vi "LINC COSMOS Item.vi"(5 "ignore":bool, 6 "ID?":bool, 8 "error in (no error)":errorcluster, 9 "packet fields":T1, 10 "packet index":i32, 11 "packets in":T2[](array[typedef])) -> (0 "error out":errorcluster, 2 "item index":i32, 3 "packets out":T2[](array[typedef]))   [LabVIEW 2018, in "STEPkgDriver_LINC.lvlib"]
uses:
  STEPkgDriver_LINC.lvlib
  LINC Format Prototype.ctl
  LINC Packet.ctl
  LINC Packet Fields.ctl
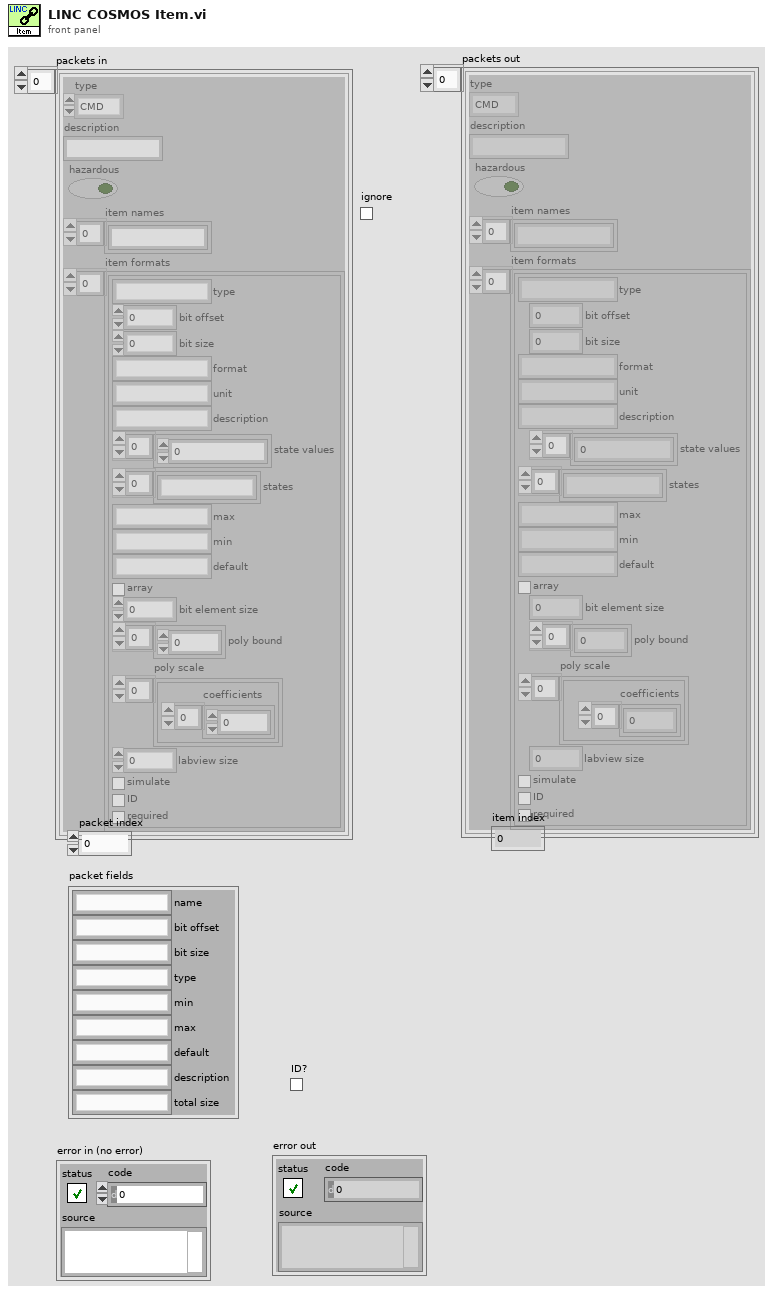
[diagram p1: front panel]
types:
  T1 = typedef "STEPkgDriver_LINC.lvlib/LINC Packet Fields.ctl" = cluster{"name":string, "bit offset":string, "bit size":string, "type":string, "min":string, "max":string, "default":string, "description":string, "total size":string}
  T2 = typedef "STEPkgDriver_LINC.lvlib/LINC Packet.ctl" = cluster{"type":enum16{"CMD", "TLM"}, "description":string, "hazardous":bool, "item names":string[], "item formats":T3[]}
  T3 = typedef "STEPkgDriver_LINC.lvlib/LINC Format Prototype.ctl" = cluster{"type":string, "bit offset":i32, "bit size":i32, "format":string, "unit":string, "description":string, "state values":i64[], "states":string[], "max":string, "min":string, "default":string, "array":bool, "bit element size":i32, "poly bound":dbl[], "poly scale":cluster{"coefficients":dbl[]}[], "labview size":i32, "simulate":bool, "ID":bool, "required":bool}
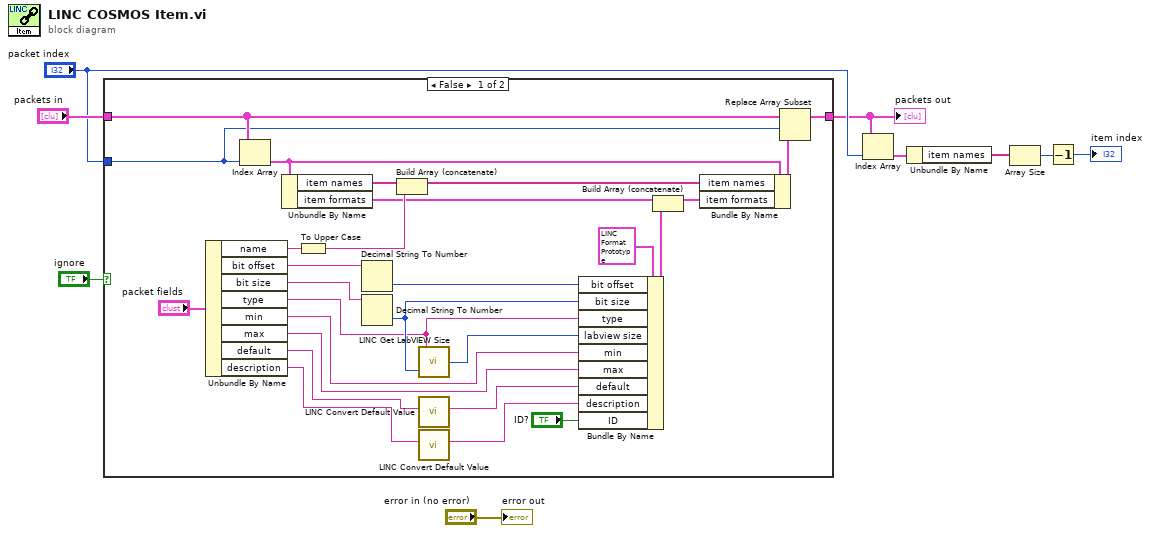
[diagram p0: block diagram]
diagram:
  n1 = case shown="False" "ignore" {
    tunnel: "packets in" -> [w21 w37]
    tunnel: [w20 w37] -> w5
    tunnel: "packet index" -> [w10 _]
    frame False {
      n2 = Unbundle By Name("packet fields") -> ("name"=w17:string, "bit offset"=w16:string, "bit size"=w15:string, "type"=w14:string, "min"=w13:string, "max"=w12:string, "default"=w11:string, "description"=w29:string)
      n3 = Index Array(array=w21, index=w10) -> (element=w27:T2)
      n4 = Unbundle By Name(w27) -> ("item names"=w25:string[], "item formats"=w22:T3[])
      n5 = To Upper Case(1:w17) -> (0:w32:string)
      n6 = Decimal String To Number(string=w16) -> (number=w33:i32)  [unwired: 2 in, 1 out]
      n7 = Decimal String To Number(string=w15) -> (number=w31:i32)  [unwired: 2 in, 1 out]
      n8 = Build Array (concatenate)(w25, w32) -> (w24:string[])
      n9 = call "LINC Get LabVIEW Size.vi"("bit size"=w31, "type"=w14) -> ("labview size"=w30:i32)
      n10 = call "LINC Convert Default Value.vi"("default in"=w11) -> ("default out"=w34:string)  [unwired: 10 in]
      n11 = call "LINC Convert Default Value.vi"("default in"=w29) -> ("default out"=w28:string)  [unwired: 10 in]
      n12 = Bundle By Name(cluster=T3 {"type"="", "bit offset"=0, "bit size"=0, "format"="", "unit"="", "description"="", "state values"=[], "states"=[], "max"="", "min"="", "default"="", "array"=FALSE, "bit element size"=0, "poly bound"=[], "poly scale"=[], "labview size"=0, "simulate"=FALSE, "ID"=FALSE, "required"=FALSE} ("data"), "bit offset"=w33, "bit size"=w31, "type"=w14, "labview size"=w30, "min"=w13, "max"=w12, "default"=w34, "description"=w28, "ID"="ID?") -> (w35:T3)
      n13 = Build Array (concatenate)(w22, w35) -> (w23:T3[])
      n14 = Bundle By Name(cluster=w27, "item names"=w24, "item formats"=w23) -> (w26:T2)
      n15 = Replace Array Subset(array=w21, new element=w26, index=w10) -> (w20:T2[])
    }
    frame True {
    }
  }
  "packets out" <- w5
  n16 = Index Array(array=w5, index="packet index") -> (element=w4:T2)
  n17 = Unbundle By Name(w4) -> ("item names"=w3:string[])
  n18 = Array Size(array=w3) -> (size(s)=w2:i32)
  n19 = Decrement(x=w2) -> (x-1=→"item index":i32)
  "error out" <- "error in (no error)"
